vi "DATAreader5.vi"(6 "manual ADC rate, kHz":dbl=625.0, 7 "data info template":refnum<vi>, 10 "Cluster":cluster{"howmany":i16, "auto/man.":bool}={"howmany"=1, "auto/man."=FALSE} {"howmany" min=1 max=2}) -> (0 "error out":errorcluster, 1 "manual ADC rate?":bool, 2 "ADC type":i32, 3 "source":T1={"data path"=["D:\\LV\\testData\\11_06_14\\10_36_14ch#1", "D:\\LV\\testData\\11_06_14\\10_36_14ch#2", "D:\\LV\\testData\\11_06_14\\10_36_14ch#3", "D:\\LV\\testData\\11_06_14\\10_36_14ch#4", "D:\\LV\\testData\\11_06_14\\10_36_14ch#5", "D:\\LV\\testData\\11_06_14\\10_36_14ch#6", "D:\\LV\\testData\\11_06_14\\10_36_14ch#7", "D:\\LV\\testData\\11_06_14\\10_36_14ch#8", "D:\\LV\\testData\\11_06_14\\10_36_14ch#9", "D:\\LV\\testData\\11_06_14\\10_36_14ch#10", "D:\\LV\\testData\\11_06_14\\10_36_14ch#11", "D:\\LV\\testData\\11_06_14\\10_36_14ch#12", "D:\\LV\\testData\\11_06_14\\10_36_14ch#13", "D:\\LV\\testData\\11_06_14\\10_36_14ch#14", "D:\\LV\\testData\\11_06_14\\10_36_14ch#15", "D:\\LV\\testData\\11_06_14\\10_36_14ch#16", "D:\\LV\\testData\\11_06_14\\10_36_14ch#17", "D:\\LV\\testData\\11_06_14\\10_36_14ch#18", "D:\\LV\\testData\\11_06_14\\10_36_14ch#19", "D:\\LV\\testData\\11_06_14\\10_36_14ch#20", "D:\\LV\\testData\\11_06_14\\10_36_14ch#21", "D:\\LV\\testData\\11_06_14\\10_36_14ch#22", "D:\\LV\\testData\\11_06_14\\10_36_14ch#23", "D:\\LV\\testData\\11_06_14\\10_36_14ch#24", "D:\\LV\\testData\\11_06_14\\10_36_14ch#25", "D:\\LV\\testData\\11_06_14\\10_36_14ch#26", "D:\\LV\\testData\\11_06_14\\10_36_14ch#27", "D:\\LV\\testData\\11_06_14\\10_36_14ch#28", "D:\\LV\\testData\\11_06_14\\10_36_14ch#29", "D:\\LV\\testData\\11_06_14\\10_36_14ch#30"], "data"=[{"t0"=timestamp(0 s since 1904-01-01), "dt"=0.00015000000000000001, "Y"=array[600 elements], "attributes"=variant("source"=variant(cluster{"data path":string, "ADCintercadr_s":dbl, "data info":cluster{"probe name":string, "signal type":string, "Unit":string, "variable":string, "amplific.":dbl, "use or not *.info.txt?":i16, "U cascade, kV":string, "attenuation":dbl, "probe area, cm2":dbl, "plasma, a.m.u.":dbl}} {"data path"="D:\\LV\\testData\\11_06_14\\10_36_14ch#1", "ADCintercadr_s"=5e-06, "data info"={"probe name"="", "signal type"="", "Unit"="", "variable"="", "amplific."=0.0, "use or not *.info.txt?"=0, "U cascade, kV"="", "attenuation"=0.0, "probe area, cm2"=0.0, "plasma, a.m.u."=0.0}}))}, {"t0"=timestamp(4.999999999999959e-06 s since 1904-01-01), "dt"=0.00015000000000000001, "Y"=array[600 elements], "attributes"=variant("source"=variant(cluster{"data path":string, "ADCintercadr_s":dbl, "data info":cluster{"probe name":string, "signal type":string, "Unit":string, "variable":string, "amplific.":dbl, "use or not *.info.txt?":i16, "U cascade, kV":string, "attenuation":dbl, "probe area, cm2":dbl, "plasma, a.m.u.":dbl}} {"data path"="D:\\LV\\testData\\11_06_14\\10_36_14ch#2", "ADCintercadr_s"=5e-06, "data info"={"probe name"="", "signal type"="", "Unit"="", "variable"="", "amplific."=0.0, "use or not *.info.txt?"=0, "U cascade, kV"="", "attenuation"=0.0, "probe area, cm2"=0.0, "plasma, a.m.u."=0.0}}))}, {"t0"=timestamp(9.999999999999972e-06 s since 1904-01-01), "dt"=0.00015000000000000001, "Y"=array[600 elements], "attributes"=variant("source"=variant(cluster{"data path":string, "ADCintercadr_s":dbl, "data info":cluster{"probe name":string, "signal type":string, "Unit":string, "variable":string, "amplific.":dbl, "use or not *.info.txt?":i16, "U cascade, kV":string, "attenuation":dbl, "probe area, cm2":dbl, "plasma, a.m.u.":dbl}} {"data path"="D:\\LV\\testData\\11_06_14\\10_36_14ch#3", "ADCintercadr_s"=5e-06, "data info"={"probe name"="", "signal type"="", "Unit"="", "variable"="", "amplific."=0.0, "use or not *.info.txt?"=0, "U cascade, kV"="", "attenuation"=0.0, "probe area, cm2"=0.0, "plasma, a.m.u."=0.0}}))}, {"t0"=timestamp(1.4999999999999985e-05 s since 1904-01-01), "dt"=0.00015000000000000001, "Y"=array[600 elements], "attributes"=variant("source"=variant(cluster{"data path":string, "ADCintercadr_s":dbl, "data info":cluster{"probe name":string, "signal type":string, "Unit":string, "variable":string, "amplific.":dbl, "use or not *.info.txt?":i16, "U cascade, kV":string, "attenuation":dbl, "probe area, cm2":dbl, "plasma, a.m.u.":dbl}} {"data path"="D:\\LV\\testData\\11_06_14\\10_36_14ch#4", "ADCintercadr_s"=5e-06, "data info"={"probe name"="", "signal type"="", "Unit"="", "variable"="", "amplific."=0.0, "use or not *.info.txt?"=0, "U cascade, kV"="", "attenuation"=0.0, "probe area, cm2"=0.0, "plasma, a.m.u."=0.0}}))}, {"t0"=timestamp(1.9999999999999998e-05 s since 1904-01-01), "dt"=0.00015000000000000001, "Y"=array[600 elements], "attributes"=variant("source"=variant(cluster{"data path":string, "ADCintercadr_s":dbl, "data info":cluster{"probe name":string, "signal type":string, "Unit":string, "variable":string, "amplific.":dbl, "use or not *.info.txt?":i16, "U cascade, kV":string, "attenuation":dbl, "probe area, cm2":dbl, "plasma, a.m.u.":dbl}} {"data path"="D:\\LV\\testData\\11_06_14\\10_36_14ch#5", "ADCintercadr_s"=5e-06, "data info"={"probe name"="", "signal type"="", "Unit"="", "variable"="", "amplific."=0.0, "use or not *.info.txt?"=0, "U cascade, kV"="", "attenuation"=0.0, "probe area, cm2"=0.0, "plasma, a.m.u."=0.0}}))}, {"t0"=timestamp(2.4999999999999957e-05 s since 1904-01-01), "dt"=0.00015000000000000001, "Y"=array[600 elements], "attributes"=variant("source"=variant(cluster{"data path":string, "ADCintercadr_s":dbl, "data info":cluster{"probe name":string, "signal type":string, "Unit":string, "variable":string, "amplific.":dbl, "use or not *.info.txt?":i16, "U cascade, kV":string, "attenuation":dbl, "probe area, cm2":dbl, "plasma, a.m.u.":dbl}} {"data path"="D:\\LV\\testData\\11_06_14\\10_36_14ch#6", "ADCintercadr_s"=5e-06, "data info"={"probe name"="", "signal type"="", "Unit"="", "variable"="", "amplific."=0.0, "use or not *.info.txt?"=0, "U cascade, kV"="", "attenuation"=0.0, "probe area, cm2"=0.0, "plasma, a.m.u."=0.0}}))}, {"t0"=timestamp(2.999999999999997e-05 s since 1904-01-01), "dt"=0.00015000000000000001, "Y"=array[600 elements], "attributes"=variant("source"=variant(cluster{"data path":string, "ADCintercadr_s":dbl, "data info":cluster{"probe name":string, "signal type":string, "Unit":string, "variable":string, "amplific.":dbl, "use or not *.info.txt?":i16, "U cascade, kV":string, "attenuation":dbl, "probe area, cm2":dbl, "plasma, a.m.u.":dbl}} {"data path"="D:\\LV\\testData\\11_06_14\\10_36_14ch#7", "ADCintercadr_s"=5e-06, "data info"={"probe name"="", "signal type"="", "Unit"="", "variable"="", "amplific."=0.0, "use or not *.info.txt?"=0, "U cascade, kV"="", "attenuation"=0.0, "probe area, cm2"=0.0, "plasma, a.m.u."=0.0}}))}, {"t0"=timestamp(3.499999999999998e-05 s since 1904-01-01), "dt"=0.00015000000000000001, "Y"=array[600 elements], "attributes"=variant("source"=variant(cluster{"data path":string, "ADCintercadr_s":dbl, "data info":cluster{"probe name":string, "signal type":string, "Unit":string, "variable":string, "amplific.":dbl, "use or not *.info.txt?":i16, "U cascade, kV":string, "attenuation":dbl, "probe area, cm2":dbl, "plasma, a.m.u.":dbl}} {"data path"="D:\\LV\\testData\\11_06_14\\10_36_14ch#8", "ADCintercadr_s"=5e-06, "data info"={"probe name"="", "signal type"="", "Unit"="", "variable"="", "amplific."=0.0, "use or not *.info.txt?"=0, "U cascade, kV"="", "attenuation"=0.0, "probe area, cm2"=0.0, "plasma, a.m.u."=0.0}}))}, {"t0"=timestamp(3.9999999999999996e-05 s since 1904-01-01), "dt"=0.00015000000000000001, "Y"=array[600 elements], "attributes"=variant("source"=variant(cluster{"data path":string, "ADCintercadr_s":dbl, "data info":cluster{"probe name":string, "signal type":string, "Unit":string, "variable":string, "amplific.":dbl, "use or not *.info.txt?":i16, "U cascade, kV":string, "attenuation":dbl, "probe area, cm2":dbl, "plasma, a.m.u.":dbl}} {"data path"="D:\\LV\\testData\\11_06_14\\10_36_14ch#9", "ADCintercadr_s"=5e-06, "data info"={"probe name"="", "signal type"="", "Unit"="", "variable"="", "amplific."=0.0, "use or not *.info.txt?"=0, "U cascade, kV"="", "attenuation"=0.0, "probe area, cm2"=0.0, "plasma, a.m.u."=0.0}}))}, {"t0"=timestamp(4.4999999999999955e-05 s since 1904-01-01), "dt"=0.00015000000000000001, "Y"=array[600 elements], "attributes"=variant("source"=variant(cluster{"data path":string, "ADCintercadr_s":dbl, "data info":cluster{"probe name":string, "signal type":string, "Unit":string, "variable":string, "amplific.":dbl, "use or not *.info.txt?":i16, "U cascade, kV":string, "attenuation":dbl, "probe area, cm2":dbl, "plasma, a.m.u.":dbl}} {"data path"="D:\\LV\\testData\\11_06_14\\10_36_14ch#10", "ADCintercadr_s"=5e-06, "data info"={"probe name"="", "signal type"="", "Unit"="", "variable"="", "amplific."=0.0, "use or not *.info.txt?"=0, "U cascade, kV"="", "attenuation"=0.0, "probe area, cm2"=0.0, "plasma, a.m.u."=0.0}}))}, {"t0"=timestamp(4.999999999999997e-05 s since 1904-01-01), "dt"=0.00015000000000000001, "Y"=array[600 elements], "attributes"=variant("source"=variant(cluster{"data path":string, "ADCintercadr_s":dbl, "data info":cluster{"probe name":string, "signal type":string, "Unit":string, "variable":string, "amplific.":dbl, "use or not *.info.txt?":i16, "U cascade, kV":string, "attenuation":dbl, "probe area, cm2":dbl, "plasma, a.m.u.":dbl}} {"data path"="D:\\LV\\testData\\11_06_14\\10_36_14ch#11", "ADCintercadr_s"=5e-06, "data info"={"probe name"="", "signal type"="", "Unit"="", "variable"="", "amplific."=0.0, "use or not *.info.txt?"=0, "U cascade, kV"="", "attenuation"=0.0, "probe area, cm2"=0.0, "plasma, a.m.u."=0.0}}))}, {"t0"=timestamp(5.499999999999998e-05 s since 1904-01-01), "dt"=0.00015000000000000001, "Y"=array[600 elements], "attributes"=variant("source"=variant(cluster{"data path":string, "ADCintercadr_s":dbl, "data info":cluster{"probe name":string, "signal type":string, "Unit":string, "variable":string, "amplific.":dbl, "use or not *.info.txt?":i16, "U cascade, kV":string, "attenuation":dbl, "probe area, cm2":dbl, "plasma, a.m.u.":dbl}} {"data path"="D:\\LV\\testData\\11_06_14\\10_36_14ch#12", "ADCintercadr_s"=5e-06, "data info"={"probe name"="", "signal type"="", "Unit"="", "variable"="", "amplific."=0.0, "use or not *.info.txt?"=0, "U cascade, kV"="", "attenuation"=0.0, "probe area, cm2"=0.0, "plasma, a.m.u."=0.0}}))}, {"t0"=timestamp(5.9999999999999995e-05 s since 1904-01-01), "dt"=0.00015000000000000001, "Y"=array[600 elements], "attributes"=variant("source"=variant(cluster{"data path":string, "ADCintercadr_s":dbl, "data info":cluster{"probe name":string, "signal type":string, "Unit":string, "variable":string, "amplific.":dbl, "use or not *.info.txt?":i16, "U cascade, kV":string, "attenuation":dbl, "probe area, cm2":dbl, "plasma, a.m.u.":dbl}} {"data path"="D:\\LV\\testData\\11_06_14\\10_36_14ch#13", "ADCintercadr_s"=5e-06, "data info"={"probe name"="", "signal type"="", "Unit"="", "variable"="", "amplific."=0.0, "use or not *.info.txt?"=0, "U cascade, kV"="", "attenuation"=0.0, "probe area, cm2"=0.0, "plasma, a.m.u."=0.0}}))}, {"t0"=timestamp(6.500000000000001e-05 s since 1904-01-01), "dt"=0.00015000000000000001, "Y"=array[600 elements], "attributes"=variant("source"=variant(cluster{"data path":string, "ADCintercadr_s":dbl, "data info":cluster{"probe name":string, "signal type":string, "Unit":string, "variable":string, "amplific.":dbl, "use or not *.info.txt?":i16, "U cascade, kV":string, "attenuation":dbl, "probe area, cm2":dbl, "plasma, a.m.u.":dbl}} {"data path"="D:\\LV\\testData\\11_06_14\\10_36_14ch#14", "ADCintercadr_s"=5e-06, "data info"={"probe name"="", "signal type"="", "Unit"="", "variable"="", "amplific."=0.0, "use or not *.info.txt?"=0, "U cascade, kV"="", "attenuation"=0.0, "probe area, cm2"=0.0, "plasma, a.m.u."=0.0}}))}, {"t0"=timestamp(6.999999999999997e-05 s since 1904-01-01), "dt"=0.00015000000000000001, "Y"=array[600 elements], "attributes"=variant("source"=variant(cluster{"data path":string, "ADCintercadr_s":dbl, "data info":cluster{"probe name":string, "signal type":string, "Unit":string, "variable":string, "amplific.":dbl, "use or not *.info.txt?":i16, "U cascade, kV":string, "attenuation":dbl, "probe area, cm2":dbl, "plasma, a.m.u.":dbl}} {"data path"="D:\\LV\\testData\\11_06_14\\10_36_14ch#15", "ADCintercadr_s"=5e-06, "data info"={"probe name"="", "signal type"="", "Unit"="", "variable"="", "amplific."=0.0, "use or not *.info.txt?"=0, "U cascade, kV"="", "attenuation"=0.0, "probe area, cm2"=0.0, "plasma, a.m.u."=0.0}}))}, {"t0"=timestamp(7.499999999999998e-05 s since 1904-01-01), "dt"=0.00015000000000000001, "Y"=array[600 elements], "attributes"=variant("source"=variant(cluster{"data path":string, "ADCintercadr_s":dbl, "data info":cluster{"probe name":string, "signal type":string, "Unit":string, "variable":string, "amplific.":dbl, "use or not *.info.txt?":i16, "U cascade, kV":string, "attenuation":dbl, "probe area, cm2":dbl, "plasma, a.m.u.":dbl}} {"data path"="D:\\LV\\testData\\11_06_14\\10_36_14ch#16", "ADCintercadr_s"=5e-06, "data info"={"probe name"="", "signal type"="", "Unit"="", "variable"="", "amplific."=0.0, "use or not *.info.txt?"=0, "U cascade, kV"="", "attenuation"=0.0, "probe area, cm2"=0.0, "plasma, a.m.u."=0.0}}))}, {"t0"=timestamp(7.999999999999999e-05 s since 1904-01-01), "dt"=0.00015000000000000001, "Y"=array[600 elements], "attributes"=variant("source"=variant(cluster{"data path":string, "ADCintercadr_s":dbl, "data info":cluster{"probe name":string, "signal type":string, "Unit":string, "variable":string, "amplific.":dbl, "use or not *.info.txt?":i16, "U cascade, kV":string, "attenuation":dbl, "probe area, cm2":dbl, "plasma, a.m.u.":dbl}} {"data path"="D:\\LV\\testData\\11_06_14\\10_36_14ch#17", "ADCintercadr_s"=5e-06, "data info"={"probe name"="", "signal type"="", "Unit"="", "variable"="", "amplific."=0.0, "use or not *.info.txt?"=0, "U cascade, kV"="", "attenuation"=0.0, "probe area, cm2"=0.0, "plasma, a.m.u."=0.0}}))}, {"t0"=timestamp(8.5e-05 s since 1904-01-01), "dt"=0.00015000000000000001, "Y"=array[600 elements], "attributes"=variant("source"=variant(cluster{"data path":string, "ADCintercadr_s":dbl, "data info":cluster{"probe name":string, "signal type":string, "Unit":string, "variable":string, "amplific.":dbl, "use or not *.info.txt?":i16, "U cascade, kV":string, "attenuation":dbl, "probe area, cm2":dbl, "plasma, a.m.u.":dbl}} {"data path"="D:\\LV\\testData\\11_06_14\\10_36_14ch#18", "ADCintercadr_s"=5e-06, "data info"={"probe name"="", "signal type"="", "Unit"="", "variable"="", "amplific."=0.0, "use or not *.info.txt?"=0, "U cascade, kV"="", "attenuation"=0.0, "probe area, cm2"=0.0, "plasma, a.m.u."=0.0}}))}, {"t0"=timestamp(8.999999999999997e-05 s since 1904-01-01), "dt"=0.00015000000000000001, "Y"=array[600 elements], "attributes"=variant("source"=variant(cluster{"data path":string, "ADCintercadr_s":dbl, "data info":cluster{"probe name":string, "signal type":string, "Unit":string, "variable":string, "amplific.":dbl, "use or not *.info.txt?":i16, "U cascade, kV":string, "attenuation":dbl, "probe area, cm2":dbl, "plasma, a.m.u.":dbl}} {"data path"="D:\\LV\\testData\\11_06_14\\10_36_14ch#19", "ADCintercadr_s"=5e-06, "data info"={"probe name"="", "signal type"="", "Unit"="", "variable"="", "amplific."=0.0, "use or not *.info.txt?"=0, "U cascade, kV"="", "attenuation"=0.0, "probe area, cm2"=0.0, "plasma, a.m.u."=0.0}}))}, {"t0"=timestamp(9.499999999999998e-05 s since 1904-01-01), "dt"=0.00015000000000000001, "Y"=array[600 elements], "attributes"=variant("source"=variant(cluster{"data path":string, "ADCintercadr_s":dbl, "data info":cluster{"probe name":string, "signal type":string, "Unit":string, "variable":string, "amplific.":dbl, "use or not *.info.txt?":i16, "U cascade, kV":string, "attenuation":dbl, "probe area, cm2":dbl, "plasma, a.m.u.":dbl}} {"data path"="D:\\LV\\testData\\11_06_14\\10_36_14ch#20", "ADCintercadr_s"=5e-06, "data info"={"probe name"="", "signal type"="", "Unit"="", "variable"="", "amplific."=0.0, "use or not *.info.txt?"=0, "U cascade, kV"="", "attenuation"=0.0, "probe area, cm2"=0.0, "plasma, a.m.u."=0.0}}))}, {"t0"=timestamp(9.999999999999999e-05 s since 1904-01-01), "dt"=0.00015000000000000001, "Y"=array[600 elements], "attributes"=variant("source"=variant(cluster{"data path":string, "ADCintercadr_s":dbl, "data info":cluster{"probe name":string, "signal type":string, "Unit":string, "variable":string, "amplific.":dbl, "use or not *.info.txt?":i16, "U cascade, kV":string, "attenuation":dbl, "probe area, cm2":dbl, "plasma, a.m.u.":dbl}} {"data path"="D:\\LV\\testData\\11_06_14\\10_36_14ch#21", "ADCintercadr_s"=5e-06, "data info"={"probe name"="", "signal type"="", "Unit"="", "variable"="", "amplific."=0.0, "use or not *.info.txt?"=0, "U cascade, kV"="", "attenuation"=0.0, "probe area, cm2"=0.0, "plasma, a.m.u."=0.0}}))}, {"t0"=timestamp(0.000105 s since 1904-01-01), "dt"=0.00015000000000000001, "Y"=array[600 elements], "attributes"=variant("source"=variant(cluster{"data path":string, "ADCintercadr_s":dbl, "data info":cluster{"probe name":string, "signal type":string, "Unit":string, "variable":string, "amplific.":dbl, "use or not *.info.txt?":i16, "U cascade, kV":string, "attenuation":dbl, "probe area, cm2":dbl, "plasma, a.m.u.":dbl}} {"data path"="D:\\LV\\testData\\11_06_14\\10_36_14ch#22", "ADCintercadr_s"=5e-06, "data info"={"probe name"="", "signal type"="", "Unit"="", "variable"="", "amplific."=0.0, "use or not *.info.txt?"=0, "U cascade, kV"="", "attenuation"=0.0, "probe area, cm2"=0.0, "plasma, a.m.u."=0.0}}))}, {"t0"=timestamp(0.00010999999999999996 s since 1904-01-01), "dt"=0.00015000000000000001, "Y"=array[600 elements], "attributes"=variant("source"=variant(cluster{"data path":string, "ADCintercadr_s":dbl, "data info":cluster{"probe name":string, "signal type":string, "Unit":string, "variable":string, "amplific.":dbl, "use or not *.info.txt?":i16, "U cascade, kV":string, "attenuation":dbl, "probe area, cm2":dbl, "plasma, a.m.u.":dbl}} {"data path"="D:\\LV\\testData\\11_06_14\\10_36_14ch#23", "ADCintercadr_s"=5e-06, "data info"={"probe name"="", "signal type"="", "Unit"="", "variable"="", "amplific."=0.0, "use or not *.info.txt?"=0, "U cascade, kV"="", "attenuation"=0.0, "probe area, cm2"=0.0, "plasma, a.m.u."=0.0}}))}, {"t0"=timestamp(0.00011499999999999998 s since 1904-01-01), "dt"=0.00015000000000000001, "Y"=array[600 elements], "attributes"=variant("source"=variant(cluster{"data path":string, "ADCintercadr_s":dbl, "data info":cluster{"probe name":string, "signal type":string, "Unit":string, "variable":string, "amplific.":dbl, "use or not *.info.txt?":i16, "U cascade, kV":string, "attenuation":dbl, "probe area, cm2":dbl, "plasma, a.m.u.":dbl}} {"data path"="D:\\LV\\testData\\11_06_14\\10_36_14ch#24", "ADCintercadr_s"=5e-06, "data info"={"probe name"="", "signal type"="", "Unit"="", "variable"="", "amplific."=0.0, "use or not *.info.txt?"=0, "U cascade, kV"="", "attenuation"=0.0, "probe area, cm2"=0.0, "plasma, a.m.u."=0.0}}))}, {"t0"=timestamp(0.00011999999999999999 s since 1904-01-01), "dt"=0.00015000000000000001, "Y"=array[600 elements], "attributes"=variant("source"=variant(cluster{"data path":string, "ADCintercadr_s":dbl, "data info":cluster{"probe name":string, "signal type":string, "Unit":string, "variable":string, "amplific.":dbl, "use or not *.info.txt?":i16, "U cascade, kV":string, "attenuation":dbl, "probe area, cm2":dbl, "plasma, a.m.u.":dbl}} {"data path"="D:\\LV\\testData\\11_06_14\\10_36_14ch#25", "ADCintercadr_s"=5e-06, "data info"={"probe name"="", "signal type"="", "Unit"="", "variable"="", "amplific."=0.0, "use or not *.info.txt?"=0, "U cascade, kV"="", "attenuation"=0.0, "probe area, cm2"=0.0, "plasma, a.m.u."=0.0}}))}, {"t0"=timestamp(0.000125 s since 1904-01-01), "dt"=0.00015000000000000001, "Y"=array[600 elements], "attributes"=variant("source"=variant(cluster{"data path":string, "ADCintercadr_s":dbl, "data info":cluster{"probe name":string, "signal type":string, "Unit":string, "variable":string, "amplific.":dbl, "use or not *.info.txt?":i16, "U cascade, kV":string, "attenuation":dbl, "probe area, cm2":dbl, "plasma, a.m.u.":dbl}} {"data path"="D:\\LV\\testData\\11_06_14\\10_36_14ch#26", "ADCintercadr_s"=5e-06, "data info"={"probe name"="", "signal type"="", "Unit"="", "variable"="", "amplific."=0.0, "use or not *.info.txt?"=0, "U cascade, kV"="", "attenuation"=0.0, "probe area, cm2"=0.0, "plasma, a.m.u."=0.0}}))}, {"t0"=timestamp(0.00013000000000000002 s since 1904-01-01), "dt"=0.00015000000000000001, "Y"=array[600 elements], "attributes"=variant("source"=variant(cluster{"data path":string, "ADCintercadr_s":dbl, "data info":cluster{"probe name":string, "signal type":string, "Unit":string, "variable":string, "amplific.":dbl, "use or not *.info.txt?":i16, "U cascade, kV":string, "attenuation":dbl, "probe area, cm2":dbl, "plasma, a.m.u.":dbl}} {"data path"="D:\\LV\\testData\\11_06_14\\10_36_14ch#27", "ADCintercadr_s"=5e-06, "data info"={"probe name"="", "signal type"="", "Unit"="", "variable"="", "amplific."=0.0, "use or not *.info.txt?"=0, "U cascade, kV"="", "attenuation"=0.0, "probe area, cm2"=0.0, "plasma, a.m.u."=0.0}}))}, {"t0"=timestamp(0.00013499999999999997 s since 1904-01-01), "dt"=0.00015000000000000001, "Y"=array[600 elements], "attributes"=variant("source"=variant(cluster{"data path":string, "ADCintercadr_s":dbl, "data info":cluster{"probe name":string, "signal type":string, "Unit":string, "variable":string, "amplific.":dbl, "use or not *.info.txt?":i16, "U cascade, kV":string, "attenuation":dbl, "probe area, cm2":dbl, "plasma, a.m.u.":dbl}} {"data path"="D:\\LV\\testData\\11_06_14\\10_36_14ch#28", "ADCintercadr_s"=5e-06, "data info"={"probe name"="", "signal type"="", "Unit"="", "variable"="", "amplific."=0.0, "use or not *.info.txt?"=0, "U cascade, kV"="", "attenuation"=0.0, "probe area, cm2"=0.0, "plasma, a.m.u."=0.0}}))}, {"t0"=timestamp(0.00014 s since 1904-01-01), "dt"=0.00015000000000000001, "Y"=array[600 elements], "attributes"=variant("source"=variant(cluster{"data path":string, "ADCintercadr_s":dbl, "data info":cluster{"probe name":string, "signal type":string, "Unit":string, "variable":string, "amplific.":dbl, "use or not *.info.txt?":i16, "U cascade, kV":string, "attenuation":dbl, "probe area, cm2":dbl, "plasma, a.m.u.":dbl}} {"data path"="D:\\LV\\testData\\11_06_14\\10_36_14ch#29", "ADCintercadr_s"=5e-06, "data info"={"probe name"="", "signal type"="", "Unit"="", "variable"="", "amplific."=0.0, "use or not *.info.txt?"=0, "U cascade, kV"="", "attenuation"=0.0, "probe area, cm2"=0.0, "plasma, a.m.u."=0.0}}))}, {"t0"=timestamp(0.000145 s since 1904-01-01), "dt"=0.00015000000000000001, "Y"=array[600 elements], "attributes"=variant("source"=variant(cluster{"data path":string, "ADCintercadr_s":dbl, "data info":cluster{"probe name":string, "signal type":string, "Unit":string, "variable":string, "amplific.":dbl, "use or not *.info.txt?":i16, "U cascade, kV":string, "attenuation":dbl, "probe area, cm2":dbl, "plasma, a.m.u.":dbl}} {"data path"="D:\\LV\\testData\\11_06_14\\10_36_14ch#30", "ADCintercadr_s"=5e-06, "data info"={"probe name"="", "signal type"="", "Unit"="", "variable"="", "amplific."=0.0, "use or not *.info.txt?"=0, "U cascade, kV"="", "attenuation"=0.0, "probe area, cm2"=0.0, "plasma, a.m.u."=0.0}}))}]}, 4 "chan.in.files":i16[](array[numeric]), 11 "ADC gain applied from *.par":bool)   [LabVIEW 2014]
uses:
  <vilib>/Waveform/WDTOps.llb/WDT Number of Waveform Samples DBL.vi
panel:
  out "txt data rate":dbl[](array[numeric])
  out "allpathes":path[](array[path])
  out "Array":string[](array[string])
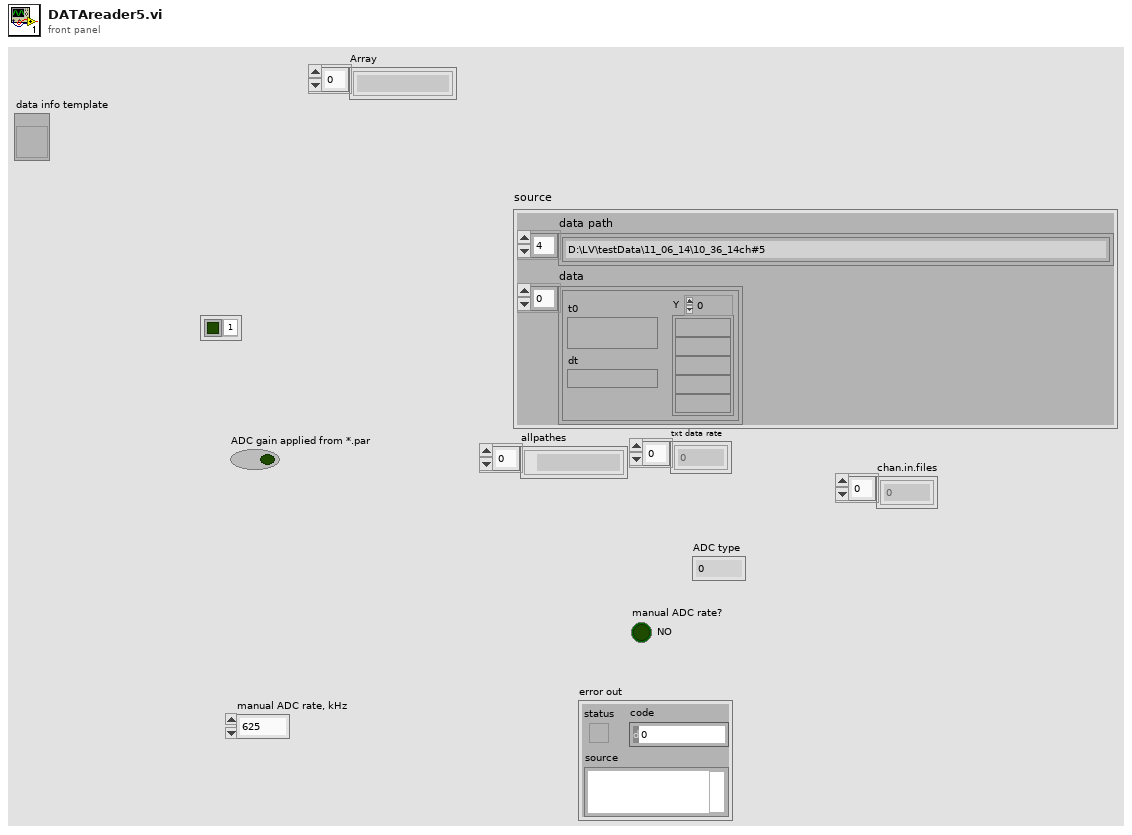
[diagram p1: front panel]
types:
  T1 = cluster{"data path":string[], "data":waveform(dbl)[]}
  T2 = enum16{"open", "replace", "create", "open or create", "replace or create", "replace or create with confirmation"}
  T3 = enum16{"deny read/write", "deny write-only", "deny none"}
  T4 = enum16{"big-endian, network order", "native, host order", "little-endian"}
  T5 = cluster{" CodeString":string, "DeviceName":string, "TimeString":string, "ChannelsMax":i16, "RealChannelsQuantity":i16, "RealKadrsQuantity":i64, "RealSamplesQuantity":i64, "TotalTime (sec) - long double in new *.par !!":string, "AdcRate (kHz)":dbl, "InterkadrDelay (ms)":dbl, "ChannelRate (kHz)":dbl, "ActiveAdcChannelArray":u32[], "AdcChannelArray":u8[], "AdcGainArray":u8[], "IsSignalArray":u8[], "DataFormat":i32, "RealKadrs64":i64, "AdcScale":dbl[], "AdcOffset":dbl[], "channel_name":string[]}
  T6 = cluster{"data path":string, "ADCintercadr_s":dbl, "data info":cluster{"use or not *.info.txt?":i16, "probe name":string, "signal type":string, "Unit":string, "variable":string, "attenuation factor":dbl, "amplification factor":dbl, "extracoef#1":dbl, "extracoef#2":dbl, "U cascade, kV":string, "probe area, cm2":dbl, "plasma, a.m.u.":dbl}, "channel_name":string, "channels_in_file":i32}
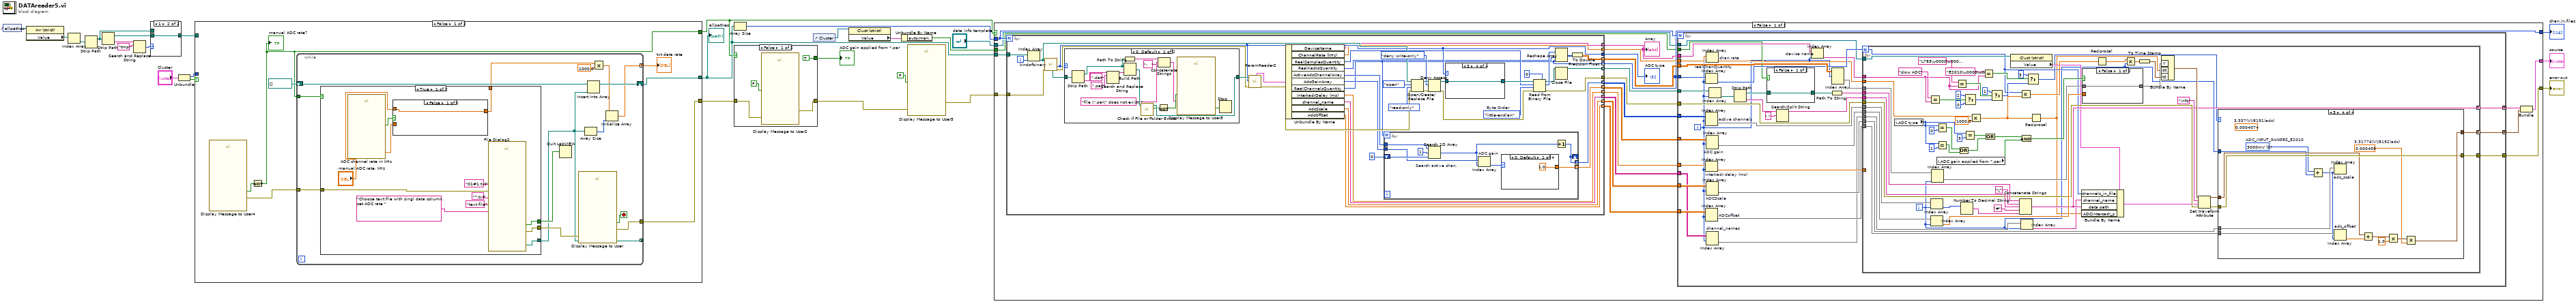
[diagram p0: block diagram]
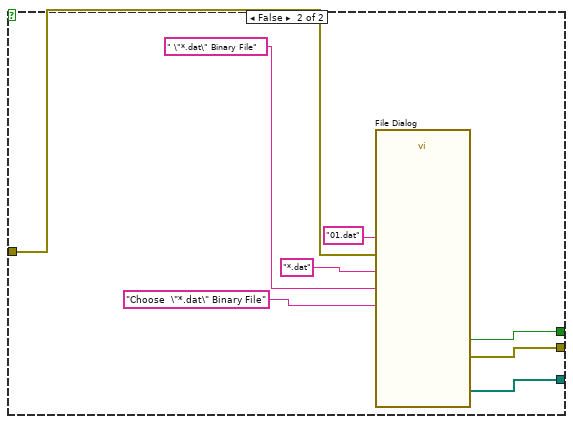
[diagram p4: hidden frame]
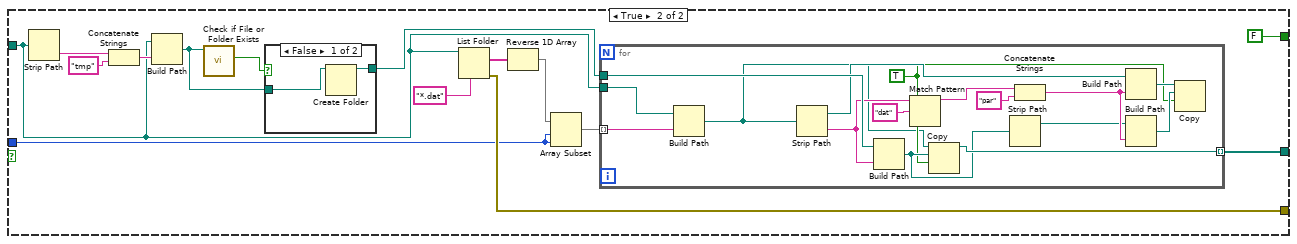
[diagram p5: hidden frame]
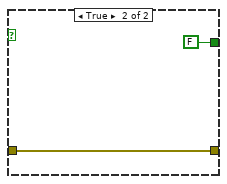
[diagram p7: hidden frame]
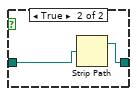
[diagram p8: hidden frame]
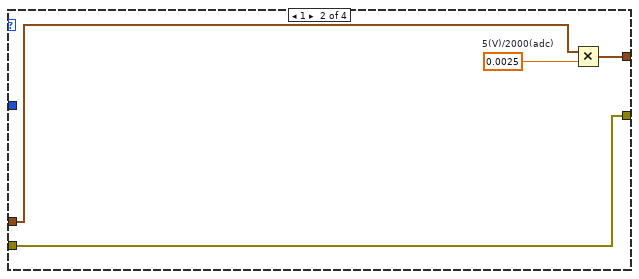
[diagram p10: hidden frame]
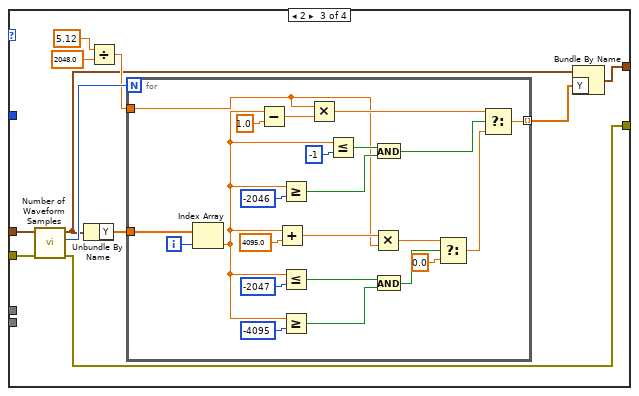
[diagram p11: hidden frame]
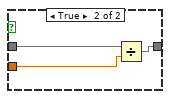
[diagram p12: hidden frame]
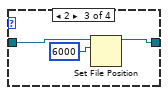
[diagram p16: hidden frame]
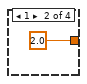
[diagram p17: hidden frame]
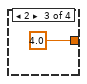
[diagram p18: hidden frame]
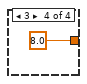
[diagram p19: hidden frame]
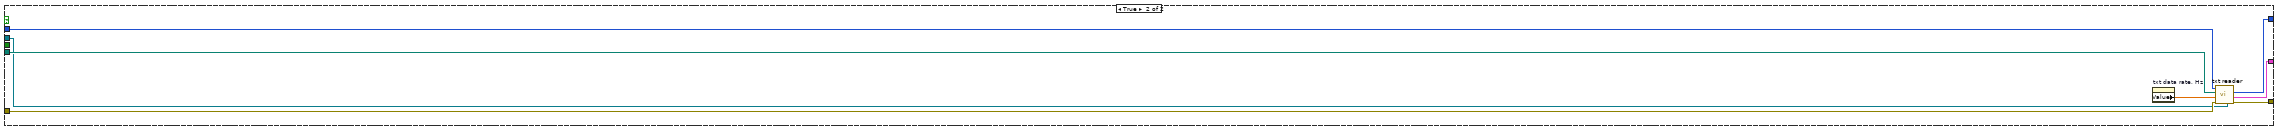
[diagram p20: hidden frame]
diagram:
  n1 = control-ref of="allpathes"() -> (w12:refnum<vi>)
  n2 = property class="Arr (strict)"(reference=w12) -> ("Value"=w11:path[])  [unwired: 1 in, 2 out]
  n3 = Index Array(array=w11) -> (element=w2:path)  [unwired: 1 in]
  n4 = Strip Path(path=w2) -> (stripped path=w5:path)  [unwired: 1 out]
  n5 = Strip Path(path=w5) -> (stripped path=w4:path, name=w7:string)
  n6 = Search and Replace String(input string=w7, search string="tmp") -> (number of replacements=w6:i32)  [unwired: 6 in, 3 out]
  n7 = case shown="1" w6 {
    tunnel: w5 -> [w28 _]
    tunnel: [w28 w29] -> w1
    tunnel: w4 -> [_ w29]
    frame 0, Default {
    }
    frame 1 {
    }
  }
  n8 = Unbundle("Cluster") -> ("howmany"=w13:i16, "auto/man."=w14:bool)
  n9 = case shown="False" w14 {
    tunnel: [w36 w76] -> w24
    tunnel: [w30 w78] -> w22
    tunnel: [w32 FALSE ("txt")] -> w18
    tunnel: w13 -> [_ w73]
    tunnel: w1 -> [_ w74]
    frame False {
      n10 = call "Display Message to User4"() -> ("error out"=w34:errorcluster, "binary"=w33:bool)  [unwired: 10 in]
      n11 = Not(x=w33) -> (.not. x?=w32:bool)
      "manual ADC rate?" <- w32
      n12 = while {
        tunnel: [w50] -> w36
        tunnel: w32 -> [w48]
        shift-right: [w47] -> w30
        shift-left: path[] [] -> [w45]
        tunnel: w34 -> [w43]
        tunnel: [w39] -> _ mode=concatenating
        tunnel: [w37] -> w31 mode=concatenating
        stop <- w44 stop-if-true
        n13 = case shown="True" w48 {
          tunnel: [w60 w69] -> w46
          tunnel: [w59 w68] -> w49
          tunnel: [w57 w66] -> w39
          tunnel: w43 -> [w55 w65]
          tunnel: [w51 _] -> w41
          frame True {
            n14 = call "ADC channel rate in kHz"() -> ("ADC channel rate, kHz"=w54:dbl, "OK"=w53:bool)  [unwired: 17 in, 1 out]
            n15 = case shown="False" w53 {
              tunnel: w54 -> [_ w64]
              tunnel: "manual ADC rate, kHz" -> [w63 _]
              tunnel: [w63 w64] -> w51
              frame False {
              }
              frame True {
              }
            }
            n16 = call "File Dialog2"("prompt"="Choose text file with singl data column, set ADC rate " ("Prompt"), "default name"="01#1.txt", "error in"=w55, "pattern (all files)"="*.txt", "pattern label"="text file" ("Prompt")) -> ("selected paths"=w57:path[], "cancelled"=w60:bool, "error out"=w59:errorcluster)  [unwired: 7 in, 1 out]
          }
          frame False {
            n17 = call "File Dialog"("prompt"="Choose  \"*.dat\" Binary File" ("Prompt"), "default name"="01.dat", "error in"=w65, "pattern (all files)"="*.dat", "pattern label"=" \"*.dat\" Binary File" ("Prompt")) -> ("selected paths"=w66:path[], "cancelled"=w69:bool, "error out"=w68:errorcluster)  [unwired: 7 in, 1 out]
          }
        }
        n18 = Quit LabVIEW(quit? (T)=w46) -> ()
        n19 = call "Display Message to User"("error in (no error)"=w49) -> ("error out"=w50:errorcluster, "NO"=w44:bool)  [unwired: 9 in]
        n20 = Array Size(array=w39) -> (size(s)=w38:i32)
        n21 = Insert Into Array(array=w45, new element=w39) -> (w47:path[])  [unwired: 1 in]
        n22 = Multiply(x=w41, y=1000.0 ("manual ADC rate, kHz")) -> (x*y=w40:dbl)
        n23 = Initialize Array(w40, w38) -> (w37:dbl[])
      }
      "txt data rate" <- w31
    }
    frame True {
      n24 = Strip Path(path=w74) -> (name=w80:string)  [unwired: 1 out]
      n25 = Concatenate Strings(w80, "tmp" ("name or relative path")) -> (w83:string)
      n26 = Build Path(base path=w74, name or relative path=w83) -> (appended path=w82:path)
      n27 = call <vilib>:"Check if File or Folder Exists.vi"("path"=w82) -> ("file or folder exists?"=w85:bool)  [unwired: 8 in, 2 out]
      n28 = case shown="False" w85 {
        tunnel: w82 -> [w105 w106]
        tunnel: [w104 w106] -> w79
        frame False {
          n29 = Create Folder(path (use dialog)=w105) -> (created path=w104:path)  [unwired: 2 in, 2 out]
        }
        frame True {
        }
      }
      n30 = List Folder(path=w74, pattern="*.dat") -> (filenames=w75:string[], error out=w76:errorcluster)  [unwired: 2 in, 2 out]
      n31 = Reverse 1D Array(array=w75) -> (reversed array=w86:string[])
      n32 = Array Subset(array=w86, index=w73, length=w73) -> (w81:string[])
      n33 = for {
        tunnel: w81 -> [w90] mode=indexing
        tunnel: w79 -> [w103]
        tunnel: [w102] -> w78 mode=indexing
        tunnel: w74 -> [w89]
        w92 = TRUE ("overwrite (F)")
        n34 = Build Path(base path=w89, name or relative path=w90) -> (appended path=w88:path)
        n35 = Strip Path(path=w88) -> (stripped path=w101:path, name=w91:string)
        n36 = Build Path(base path=w103, name or relative path=w91) -> (appended path=w99:path)
        n37 = Match Pattern(string=w91, regular expression="dat") -> (before substring=w97:string)  [unwired: 1 in, 3 out]
        n38 = Copy(9:w92, 10:w99, 11:w88) -> (3:w102:path)  [unwired: 2 in, 2 out]
        n39 = Strip Path(path=w99) -> (stripped path=w94:path)  [unwired: 1 out]
        n40 = Concatenate Strings(w97, "par" ("name or relative path")) -> (w95:string)
        n41 = Build Path(base path=w101, name or relative path=w95) -> (appended path=w100:path)
        n42 = Build Path(base path=w94, name or relative path=w95) -> (appended path=w93:path)
        n43 = Copy(9:w92, 10:w93, 11:w100) -> ()  [unwired: 2 in, 3 out]
      }
    }
  }
  "allpathes" <- w22
  n44 = Array Size(array=w22) -> (size(s)=w26:i32)
  n45 = case shown="False" w18 {
    tunnel: [TRUE FALSE ("YES")] -> w20
    tunnel: w24 -> [w110 w111]
    tunnel: [w109 w111] -> w23
    frame False {
      n46 = call "Display Message to User2"("error in (no error)"=w110, "Enable"=FALSE) -> ("error out"=w109:errorcluster)  [unwired: 8 in, 1 out]
    }
    frame True {
    }
  }
  "ADC gain applied from *.par" <- w20
  n47 = control-ref of="Cluster"() -> (w10:refnum<vi>)
  n48 = property class="Clust (strict)"(reference=w10) -> ("Value"=w9:cluster{"howmany":i16, "auto/man.":bool})  [unwired: 1 in, 2 out]
  n49 = Unbundle By Name(w9) -> ("auto/man."=w8:bool)
  n50 = call "Display Message to User3"("error in (no error)"=w23, "Enable"=FALSE ("YES")) -> ("error out"=w25:errorcluster)  [unwired: 8 in, 1 out]
  n51 = case shown="False" w18 {
    tunnel: [w134 w370] -> w27
    tunnel: w22 -> [w133 w372]
    tunnel: w26 -> [w132 w373]
    tunnel: w25 -> [w125 w371]
    tunnel: [w120 w369] -> w19
    tunnel: "data info template" -> [w118 w368]
    tunnel: [w116 w367] -> w16
    tunnel: w8 -> [w115 _]
    frame False {
      n52 = for {
        N: w132 -> [_]
        tunnel: w125 -> [w306]
        tunnel: [w296] -> w116 mode=indexing
        tunnel: [w321] -> w126 mode=indexing
        tunnel: [w301] -> w127 mode=indexing
        tunnel: w133 -> [w320]
        tunnel: [w314] -> w128 mode=indexing
        tunnel: [w310] -> w129 mode=indexing
        tunnel: [w317] -> w131
        tunnel: [w316] -> w130 mode=indexing
        tunnel: [w304] -> w124
        tunnel: [w295] -> w123 mode=indexing
        tunnel: [w294] -> w119 mode=indexing
        tunnel: [w302] -> w117 mode=indexing
        tunnel: [w293] -> w114 mode=indexing
        tunnel: [w292] -> w113 mode=indexing
        i -> [w319]
        w330 = T4."little-endian"  # Byte Order
        n53 = Index Array(array=w320, index=w319) -> (element=w309:path)
        n54 = call "kindofbinary.vi"("error in (no error)"=w306, "selected \"*.dat\" path"=w309) -> ("error out"=w305:errorcluster, "what kind of binary"=w304:i32, "output path"=w308:path)  [unwired: 7 in]
        n55 = case shown="0, Default" w304 {
          tunnel: w308 -> [w342 w347]
          tunnel: [w341 w347] -> w307
          frame 0, Default {
            n56 = Strip Path(path=w342) -> (stripped path=w333:path, name=w346:string)
            n57 = Search and Replace String(input string=w346, search string=".dat", replace string=".par" ("replace string (\"\")")) -> (result string=w343:string)  [unwired: 5 in, 3 out]
            n58 = Path To String(path=w333) -> (string=w337:string)
            n59 = Build Path(base path=w333, name or relative path=w343) -> (appended path=w338:path)
            n60 = call <vilib>:"Check if File or Folder Exists.vi"("path"=w338) -> ("file or folder exists?"=w340:bool, "dup path"=w341:path)  [unwired: 8 in, 1 out]
            n61 = Not(x=w340) -> (.not. x?=w339:bool)
            n62 = Concatenate Strings(w337, ":   " ("string"), "file \".par\" does not exist !" ("string")) -> (w334:string)
            n63 = call "Display Message to User5"("Enable"=w339, "Message"=w334) -> ("OK"=w332:bool)  [unwired: 8 in, 1 out]
            n64 = Stop(stop? (T)=w332) -> ()
          }
          frame 2 {
          }
        }
        n65 = call "ParamReader2.vi"("error in (no error)"=w305, "what kind of binary"=w304, "selected path"=w307) -> ("error out"=w313:errorcluster, "Cluster"=w303:T5)  [unwired: 6 in, 1 out]
        n66 = Unbundle By Name(w303) -> ("DeviceName"=w302:string, "ChannelRate (kHz)"=w301:dbl, "RealSamplesQuantity"=w300:i64, "RealKadrsQuantity"=w299:i64, "ActiveAdcChannelArray"=w298:u32[], "AdcGainArray"=w297:u8[], "RealChannelsQuantity"=w296:i16, "InterkadrDelay (ms)"=w295:dbl, "channel_name"=w294:string[], "AdcScale"=w293:dbl[], "AdcOffset"=w292:dbl[])
        n67 = for {
          N: w296 -> [_]
          tunnel: w298 -> [w361]
          shift-right: [w354] -> _
          shift-left: 0 -> [w359]
          tunnel: w297 -> [w358]
          tunnel: [w356] -> w316 mode=indexing
          tunnel: [w354] -> w310 mode=indexing
          n68 = Search 1D Array "Search active chan."(1D array=w361, element=1, start index (0)=w359) -> (index of element=w355:i32)
          n69 = Index Array "ADC gain"(array=w358, index=w355) -> (element=w357:u8)
          n70 = case shown="0, Default" w357 {
            tunnel: [1.0 2.0 4.0 8.0] -> w356
            frame 0, Default {
            }
            frame 1 {
            }
            frame 2 {
            }
            frame 3 {
            }
          }
          n71 = Increment(x=w355) -> (x+1=w354:i32)
        }
        n72 = Open/Create/Replace File(file path (use dialog)=w309, error in=w313, operation (0:open)=T2."open", access (0:read/write)=enum16{"read/write", "read-only", "write-only"}."read-only") -> (refnum out=w328:refnum<file>, error out=w329:errorcluster)  [unwired: 2 in, 1 out]
        n73 = Deny Access(4:w329, 6:T3."deny write-only" ("deny mode (0:deny read/write)"), 7:w328) -> (0:w325:errorcluster, 3:w312:refnum<file>)
        n74 = case shown="3" w304 {
          tunnel: w312 -> [w348 w349 w351 w353]
          tunnel: [w348 w349 w350 w353] -> w311
          frame 0, Default {
          }
          frame 1 {
          }
          frame 2 {
            n75 = Set File Position(offset (in bytes) (0)=i64 6000, refnum=w351) -> (refnum out=w350:refnum<file>)  [unwired: 2 in, 1 out]
          }
          frame 3 {
          }
        }
        n76 = Read from Binary File(5:i16 0 ("count (1)"), 8:w325, 9:w330, 10:w300, 11:w311) -> (0:w317:errorcluster, 2:w323:i16[], 3:w315:refnum<file>)  [unwired: 1 in, 1 out]
        n77 = Reshape Array(w323, w299, w296) -> (w322:i16[][])
        n78 = Close File(refnum=w315) -> (path=w314:path)  [unwired: 1 in, 1 out]
        n79 = To Double Precision Float(number=w322) -> (double precision float=w321:dbl[][])
      }
      "ADC type" <- w124
      "Array" <- w117
      n80 = for {
        N: w132 -> [_]
        tunnel: w116 -> [w166]
        tunnel: w126 -> [w168]
        tunnel: w127 -> [w169]
        tunnel: w128 -> [w165]
        tunnel: w129 -> [w164]
        tunnel: w130 -> [w163]
        tunnel: [w161] -> w134
        tunnel: w131 -> [w160]
        tunnel: w123 -> [w154]
        tunnel: [w151] -> w121 mode=concatenating
        tunnel: [w150] -> w122 mode=concatenating
        tunnel: w119 -> [w137]
        tunnel: w118 -> [w147]
        tunnel: w117 -> [w146]
        tunnel: w115 -> [w144]
        tunnel: w114 -> [w141]
        tunnel: w113 -> [w140]
        i -> [w135]
        n81 = Index Array "realChanQuantity"(array=w166, index=w135) -> (element=w149:i16)
        n82 = Index Array "active channels"(array=w164, index (row)=w135) -> (element=w159:i32[])  [unwired: 1 in]
        n83 = Index Array "interkadr delay (ms)"(array=w154, index=w135) -> (element=w153:dbl)
        n84 = Index Array "ADCoffset"(array=w140, index (row)=w135) -> (element=w138:dbl[])  [unwired: 1 in]
        n85 = Index Array "chan.rate"(array=w169, index=w135) -> (element=w148:dbl)
        n86 = Index Array "ADCScale"(array=w141, index (row)=w135) -> (element=w139:dbl[])  [unwired: 1 in]
        n87 = Index Array "ADC gain"(array=w163, index (row)=w135) -> (element=w162:dbl[])  [unwired: 1 in]
        n88 = Index Array "channel_names"(array=w137, index (row)=w135) -> (element=w136:string[])  [unwired: 1 in]
        n89 = Index Array(array=w165, index=w135) -> (element=w158:path)
        n90 = Strip Path(path=w158) -> (stripped path=w143:path, name=w156:string)
        n91 = case shown="False" w144 {
          tunnel: w143 -> [w170 w172]
          tunnel: [w170 w171] -> w142
          frame False {
          }
          frame True {
            n92 = Strip Path(path=w172) -> (stripped path=w171:path)  [unwired: 1 out]
          }
        }
        n93 = Search/Split String(string=w156, search string/char (-)="." ("regular expression")) -> (substring before match=w155:string)  [unwired: 1 in, 2 out]
        n94 = Index Array "device name"(array=w146, index=w135) -> (element=w145:string)
        n95 = Path To String(path=w142) -> (string=w152:string)
        n96 = Index Array(array=w168, index (dim 0)=w135) -> (element=w167:dbl[][])  [unwired: 2 in]
        n97 = for {
          N: w149 -> [w178]
          tunnel: w167 -> [w234]
          tunnel: w148 -> [w177]
          tunnel: w162 -> [w232]
          tunnel: [w217] -> w161
          tunnel: w160 -> [w219]
          tunnel: w159 -> [w229]
          tunnel: w152 -> [w226]
          tunnel: w155 -> [w228]
          tunnel: w153 -> [_]
          tunnel: [w208] -> w150 mode=indexing
          tunnel: [w209] -> w151 mode=indexing
          tunnel: w136 -> [w197]
          tunnel: w147 -> [w194]
          tunnel: w145 -> [w184]
          tunnel: w139 -> [w175]
          tunnel: w138 -> [w174]
          i -> [w173]
          n98 = local read "ADC type"() -> (w193:i32)
          n99 = Equal?(x="slow ADC", y=w184) -> (x = y?=w183:bool)
          n100 = Index Array(array=w229, index=w173) -> (element=w216:i32)
          n101 = Index Array(array=w232, index=w173) -> (element=w231:dbl)
          n102 = Index Array(array=w234, index (col)=w173) -> (element=w230:dbl[])  [unwired: 1 in]
          n103 = Equal?(x=w193, y=0) -> (x = y?=w214:bool)
          n104 = Equal?(x=w193, y=1) -> (x = y?=w212:bool)
          n105 = local read "ADC gain applied from *.par"() -> (w211:bool)
          n106 = Equal?(x="L783\u0000\u0000\u0000\u0000\u0000\u0000\u0000\u0000\u0000\u0000\u0000\u0000\u0000", y=w184) -> (x = y?=w187:bool)
          n107 = Or(x=w214, y=w212) -> (x .or. y?=w199:bool)
          n108 = Number To Decimal String(number=w216) -> (decimal integer string=w227:string)  [unwired: 1 in]
          n109 = Equal?(x=w193, y=3) -> (x = y?=w200:bool)
          n110 = Select(t=2, s=w183, f=0) -> (s? t:f=w181:i32)
          n111 = Multiply(x=w177, y=1000.0) -> (x*y=w204:dbl)
          n112 = Equal?(x="E2010\u0000\u0000\u0000\u0000\u0000\u0000\u0000\u0000\u0000\u0000\u0000\u0000", y=w184) -> (x = y?=w190:bool)
          n113 = Or(x=w200, y=w199) -> (x .or. y?=w198:bool)
          n114 = Select(t=1, s=w187, f=w181) -> (s? t:f=w180:i32)
          n115 = property on="Property Node" class="Clust (strict)"(reference=w194) -> ("Value"=w195:T6)  [unwired: 1 in, 2 out]
          n116 = Concatenate Strings(w226, "\\" ("string"), w228, "#" ("string"), w227) -> (w208:string)
          n117 = Multiply(x=w178, y=w204) -> (x*y=w203:dbl)
          n118 = And(x=w198, y=w211) -> (x .and. y?=w210:bool)
          n119 = Index Array(array=w197, index=w173) -> (element=w196:string)
          n120 = Select(t=3, s=w190, f=w180) -> (s? t:f=w189:i32)
          n121 = Reciprocal(x=w204) -> (1/x=w176:dbl)
          n122 = Bundle By Name(cluster=w195, "channels_in_file"=w178, "channel_name"=w196, "data path"=w208, "ADCintercadr_s"=w176) -> (w207:T6)
          n123 = case shown="False" w210 {
            tunnel: w231 -> [_ w291]
            tunnel: [w288 w290] -> w220
            tunnel: w230 -> [w288 w289]
            frame False {
            }
            frame True {
              n124 = Divide(x=w289, y=w291) -> (x/y=w290:dbl[])
            }
          }
          n125 = Reciprocal(x=w203) -> (1/x=w202:dbl)
          n126 = Multiply(x=w202, y=w173) -> (x*y=w221:dbl)
          n127 = To Time Stamp(1:w221) -> (0:w222:timestamp)
          n128 = Bundle By Name("Y"=w220, "dt"=w176, "t0"=w222) -> (w218:waveform(dbl))  [unwired: 1 in]
          n129 = Set Waveform Attribute(4:w219, 5:w207, 6:"info" ("name"), 7:w218) -> (0:w223:errorcluster, 3:w206:waveform(dbl))  [unwired: 1 out]
          n130 = case shown="3" w189 {
            tunnel: w206 -> [w235 w239 w251 w285]
            tunnel: [w235 w238 w242 w287] -> w209
            tunnel: w223 -> [w236 w237 w250 w286]
            tunnel: [w236 w237 w241 w286] -> w217
            tunnel: w175 -> [_ _ _ w281]
            tunnel: w174 -> [_ _ _ w280]
            tunnel: w173 -> [_ _ _ w277]
            frame 0, Default {
            }
            frame 1 {
              w240 = 0.0025  # 5(V)/2000(adc)
              n131 = Multiply(x=w239, y=w240) -> (x*y=w238:waveform(dbl))
            }
            frame 2 {
              n132 = call-poly <vilib>:"Number of Waveform Samples.vi"("error in (no error)"=w250, "waveform in"=w251) -> ("error out"=w241:errorcluster, "number of samples"=w249:i32, "waveform out"=w243:waveform(dbl))  [unwired: 7 in]
              n133 = Unbundle By Name(w243) -> ("Y"=w248:dbl[])
              n134 = Divide(x=5.12, y=2048.0) -> (x/y=w245:dbl)
              n135 = for {
                N: w249 -> [_]
                tunnel: w248 -> [w273]
                tunnel: w245 -> [w255]
                tunnel: [w252] -> w244 mode=indexing
                i -> [w272]
                n136 = Index Array(array=w273, index=w272) -> (element=w258:dbl)
                n137 = Subtract(x=w258, y=1.0) -> (x-y=w266:dbl)
                n138 = Add(x=w258, y=4095.0) -> (x+y=w256:dbl)
                n139 = Greater Or Equal?(x=w258, y=i16 -2046) -> (x >= y?=w271:bool)
                n140 = Less Or Equal?(x=w258, y=i16 -2047 ("length")) -> (x <= y?=w265:bool)
                n141 = Greater Or Equal?(x=w258, y=i16 -4095) -> (x >= y?=w264:bool)
                n142 = Multiply(x=w255, y=w266) -> (x*y=w257:dbl)
                n143 = Less Or Equal?(x=w258, y=i16 -1 ("length")) -> (x <= y?=w274:bool)
                n144 = Multiply(x=w256, y=w255) -> (x*y=w254:dbl)
                n145 = And(x=w274, y=w271) -> (x .and. y?=w267:bool)
                n146 = And(x=w265, y=w264) -> (x .and. y?=w261:bool)
                n147 = Select(t=w254, s=w261, f=0.0) -> (s? t:f=w260:dbl)
                n148 = Select(t=w257, s=w267, f=w260) -> (s? t:f=w252:dbl)
              }
              n149 = Bundle By Name(cluster=w243, "Y"=w244) -> (w242:waveform(dbl))
            }
            frame 3 {
              w279 = u16 0 items=["3000mV", "1000mV", "300mV"]  # ADC_INPUT_RANGES_E2010
              w282 = 0.000405  # 3.31776(V)/8192(adc)
              (unwired) 0.0004074  # 3.337(V)/8191(adc)
              n150 = Add(x=w279, y=w277) -> (x+y=w276:i32)
              n151 = Index Array "adc_scale"(array=w281, index=w276) -> ()  [unwired: 1 out]
              n152 = Index Array "adc_offset"(array=w280, index=w276) -> (element=w278:dbl)
              n153 = Add(x=w285, y=w278) -> (x+y=w284:waveform(dbl))
              n154 = Multiply(x=w284, y=1.0) -> (x*y=w283:waveform(dbl))
              n155 = Multiply(x=w283, y=w282) -> (x*y=w287:waveform(dbl))
            }
          }
        }
      }
      n156 = Bundle(w122, w121) -> (w120:cluster{string[], waveform(dbl)[]})  [unwired: 1 in]
    }
    frame True {
      n157 = property on="txt data rate, Hz" class="Arr (strict)"() -> ("Value"=w366:dbl[])  [unwired: 2 in, 2 out]
      n158 = call "txt reader.vi"("data info template"=w368, "error in (no error)"=w371, "sampling rate, Hz"=w366, "file paths"=w372, "how many files"=w373) -> ("error out"=w370:errorcluster, "source txt"=w369:T1, "channels quantity in file"=w367:i32[])  [unwired: 3 in, 1 out]
    }
  }
  "error out" <- w27
  "source" <- w19
  "chan.in.files" <- w16
